vi "cam0-制作槽边选框ROI-2.vi"(6 "槽形状参数配置":cluster{"槽形态半长":sgl, "槽形态半宽":sgl}={"槽形态半长"=50.0, "槽形态半宽"=20.0}, 8 "产品位指向角度":sgl, 9 "槽宽":sgl, 10 "槽点位":cluster{"X":sgl, "Y":sgl}, 11 "Cut基点":cluster{"X":sgl, "Y":sgl}) -> (1 "ROI槽区":T1 {"Contours"."Type" items=["No Selection", "Point", "Line", "Rectangle", "Oval", "Polygon", "Freehand Region", "Annulus", "Unused2", "Unused3", "Broken Line", "Freehand Line", "Rotated Rectangle"]}, 2 "ROI槽边白条区域":T1 {"Contours"."Type" items=["No Selection", "Point", "Line", "Rectangle", "Oval", "Polygon", "Freehand Region", "Annulus", "Unused2", "Unused3", "Broken Line", "Freehand Line", "Rotated Rectangle"]})   [LabVIEW 2018]
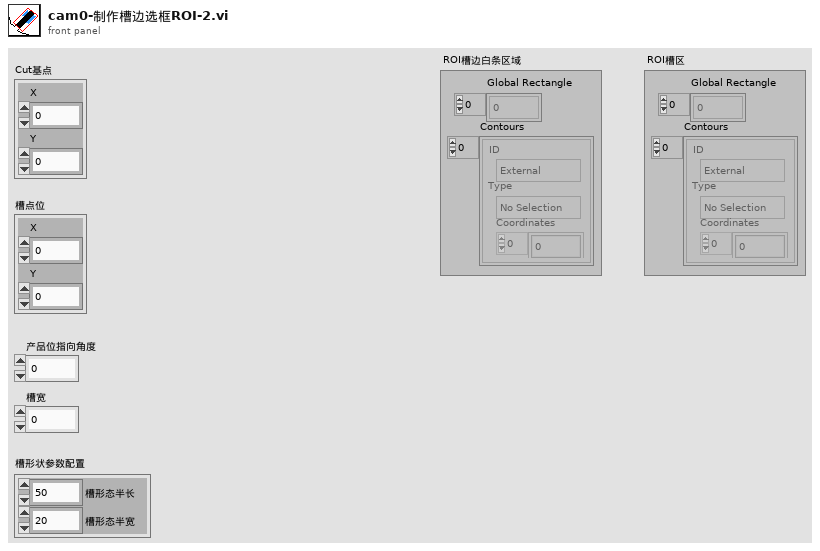
[diagram p1: front panel]
types:
  T1 = typedef "ROI Descriptor" = cluster{"Global Rectangle":i32[], "Contours":cluster{"ID":enum32{"External", "Internal"}, "Type":u32, "Coordinates":i32[]}[]}
  T2 = typedef "IMAQ Rectangle" = cluster{"Left":i32, "Top":i32, "Right":i32, "Bottom":i32, "Rotation":dbl}
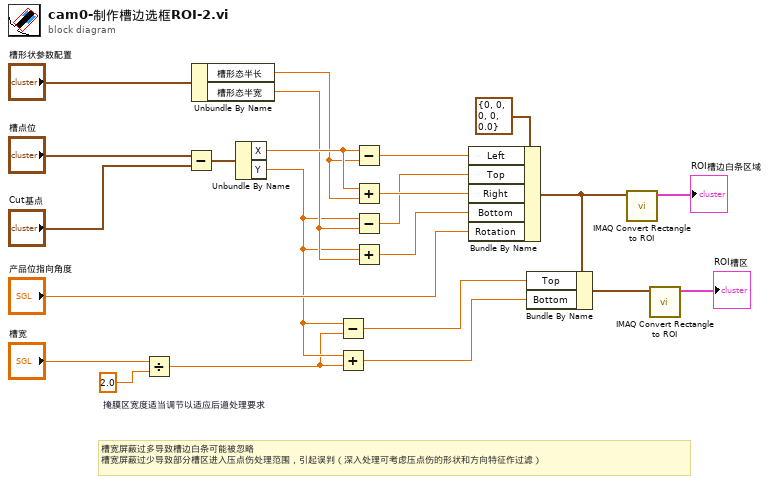
[diagram p0: block diagram]
diagram:
  w3 = sgl 2.0  # 掩膜区宽度适当调节以适应后道处理要求
  # "槽宽屏蔽过多导致槽边白条可能被忽略\n槽宽屏蔽过少导致部分槽区进入压点伤处理范围，引起误判（深入处理可考虑压点伤的形状和方向特征作过滤）"
  n1 = Divide(x="槽宽", y=w3) -> (x/y=w1:sgl)
  n2 = Subtract(x="槽点位", y="Cut基点") -> (x-y=w23:cluster{"X":sgl, "Y":sgl})
  n3 = Unbundle By Name("槽形状参数配置") -> ("槽形态半长"=w12:sgl, "槽形态半宽"=w11:sgl)
  n4 = Unbundle By Name(w23) -> ("X"=w18:sgl, "Y"=w8:sgl)
  n5 = Subtract(x=w8, y=w1) -> (x-y=w7:sgl)
  n6 = Add(x=w8, y=w1) -> (x+y=w6:sgl)
  n7 = Subtract(x=w18, y=w12) -> (x-y=w19:sgl)
  n8 = Add(x=w18, y=w12) -> (x+y=w21:sgl)
  n9 = Subtract(x=w8, y=w11) -> (x-y=w20:sgl)
  n10 = Add(x=w8, y=w11) -> (x+y=w22:sgl)
  n11 = Bundle By Name(cluster=T2 {"Left"=0, "Top"=0, "Right"=0, "Bottom"=0, "Rotation"=0.0} ("Rectangle"), "Left"=w19, "Top"=w20, "Right"=w21, "Bottom"=w22, "Rotation"="产品位指向角度") -> (w9:T2)
  n12 = Bundle By Name(cluster=w9, "Top"=w7, "Bottom"=w6) -> (w5:T2)
  n13 = call "IMAQ Convert Rectangle to ROI"("Rectangle"=w9) -> ("ROI Descriptor"=→"ROI槽边白条区域":T1)  [unwired: 8 in, 1 out]
  n14 = call "IMAQ Convert Rectangle to ROI"("Rectangle"=w5) -> ("ROI Descriptor"=→"ROI槽区":T1)  [unwired: 8 in, 1 out]
